vi "RETURN ITEM FRONT PANEL.vi"(9 "Main State":refnum<vi>, 10 "USER/ITEM DATA TRANSFER":refnum<vi>, 11 "RETURN ITEM":refnum<vi>) -> ()   [LabVIEW 2019]
uses:
  Controls/Table Data Types/Inventory Data Type.ctl
  <vilib>/addons/database/Auxilliary.llb/DB Tools Cursor Type.ctl
  Controls/Table Data Types/User Data Type.ctl
  Controls/State Variables/Main States.ctl
  Controls/Table Data Types/Checked In Archive Data Type.ctl
  Controls/Column Names/Inventory Column Names.ctl
  <vilib>/addons/database/Connection.llb/DB Tools Open Connec (String).vi
  <vilib>/addons/database/Connection.llb/Conn Execute.vi
  <vilib>/addons/database/Recordset.llb/Rec Fetch Recordset Data (R).vi
  <vilib>/addons/database/Recordset.llb/Rec Destroy - Connection.vi
  <vilib>/addons/database/_DB Variant To Data/Database Variant To Data.xnode
  <vilib>/addons/database/NI_Database_API.lvlib
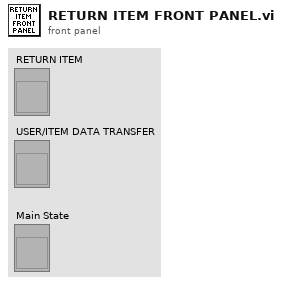
[diagram p1: front panel]
types:
  T1 = typedef "NI_Database_API.lvlib/DB Tools Cursor Type.ctl" = enum16{"forward-only", "keyset", "dynamic", "static"}
  T2 = typedef "Inventory Data Type.ctl" = cluster{"Identifier":string, "BYU ICN #":string, "Item Description":string, "Comments":string, "Checked Out Date":string, "Due Date":string, "Check Out Location":string, "Reminder Count":i32, "Most Recent Reminder Date":string, "BYU ID #":string, "Building/Room":string, "Location in Room":string, "Manual":string, "Manufacturer":string, "Model #":string, "Serial #":string, "Date Acquired":string}
  T3 = typedef "User Data Type.ctl" = cluster{"BYU ID #":string, "First Name":string, "Last Name":string, "Phone Number":string, "Email":string, "Department":string, "Graduation Status":string, "Anticipated Graduation Year":string, "Credit Score":dbl, "Date Added":string, "Graduation Clearance Date":string, "Picture File Name":string, "User Comments":string}
  T4 = typedef "Main States.ctl" = enum16{"INIT", "IDLE", "ADD USER", "EDIT USER", "ADD ITEM", "EDIT ITEM", "RETURN ITEMS", "SEARCH DATABASE", "USER ITEMS", "EDIT ITEMS", "CHECK OUT ITEMS", "TRANSFER ITEMS", "PSC SALES", "ATRIUM", "INVENTORY TRACKING", "SETTINGS", "REMINDER EMAILS", "END"}
  T5 = cluster{"DATA TYPE":enum16{"BYU ID", "ME#/IDENTIFIER", "BYU ICN"}, "DATA":string}
  T6 = typedef "Inventory Column Names.ctl" = string[]
  T7 = typedef "Checked In Archive Data Type.ctl" = cluster{"Identifier":string, "BYU ICN #":string, "Item Description":string, "Comments":string, "Checked Out Date":string, "Due Date":string, "Check Out Location":string, "Reminder Count":i32, "Most Recent Reminder Date":string, "BYU ID #":string, "Building/Room":string, "Location in Room":string, "Manual":string, "Manufacturer":string, "Model #":string, "Serial #":string, "Date Acquired":string, "Date Returned":string}
  T8 = typedef "NI_Database_API.lvlib/Conn ObjectReference.ctl" = refnum<k1>
  T9 = typedef "NI_Database_API.lvlib/Rec ObjectReference.ctl" = refnum<k1>
  T10 = cluster{"DATA TYPE":enum16{"BYU ID", "ME#/IDENTIFIER", "BYU ICN"}, "DATA":string}[]
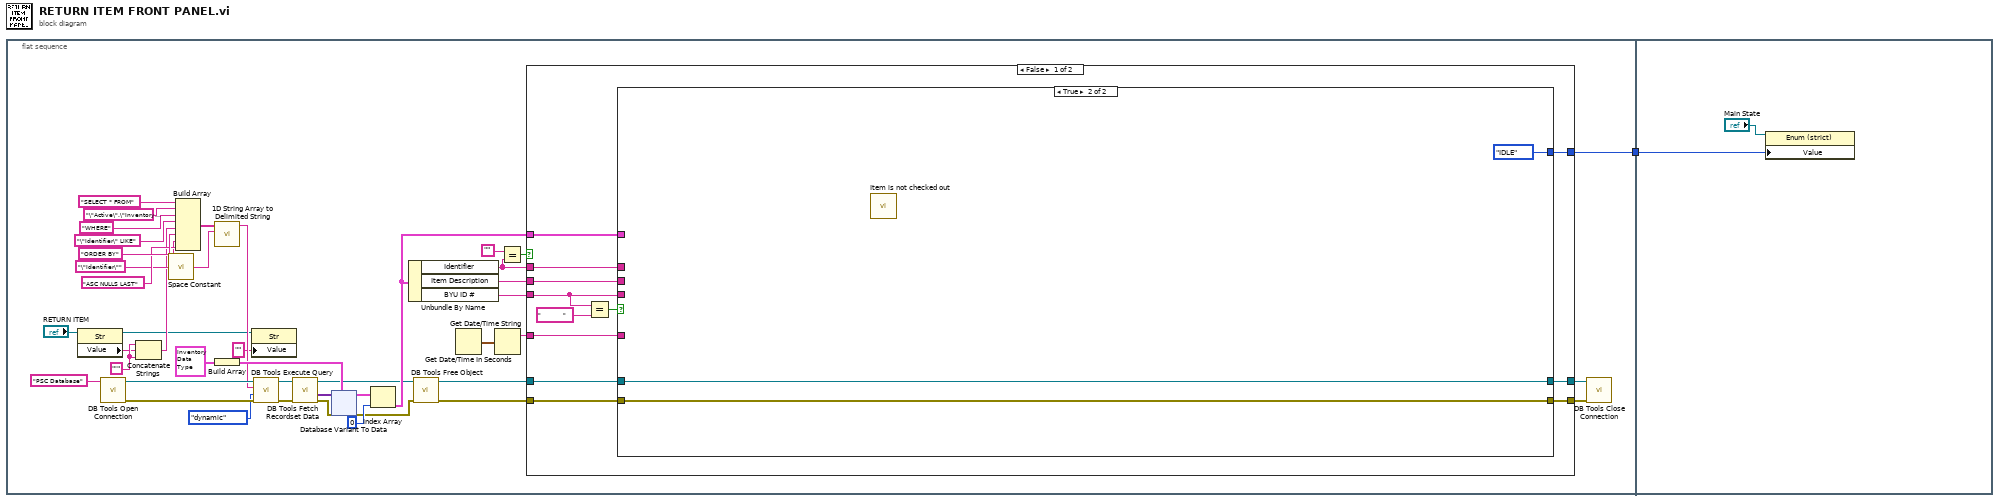
[diagram p0: block diagram]
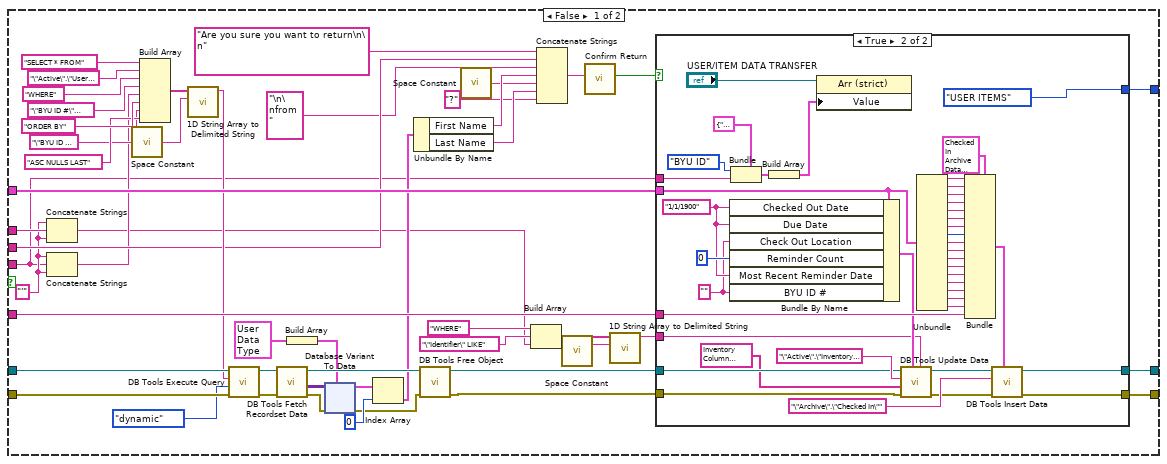
[diagram p2: hidden frame]
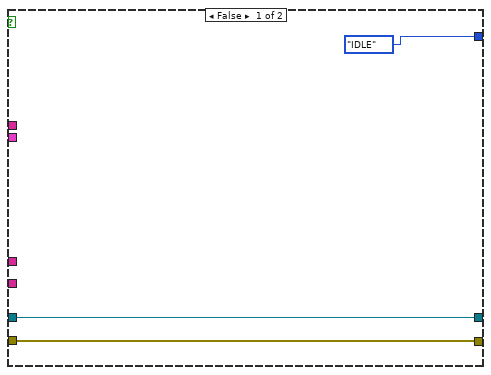
[diagram p3: hidden frame]
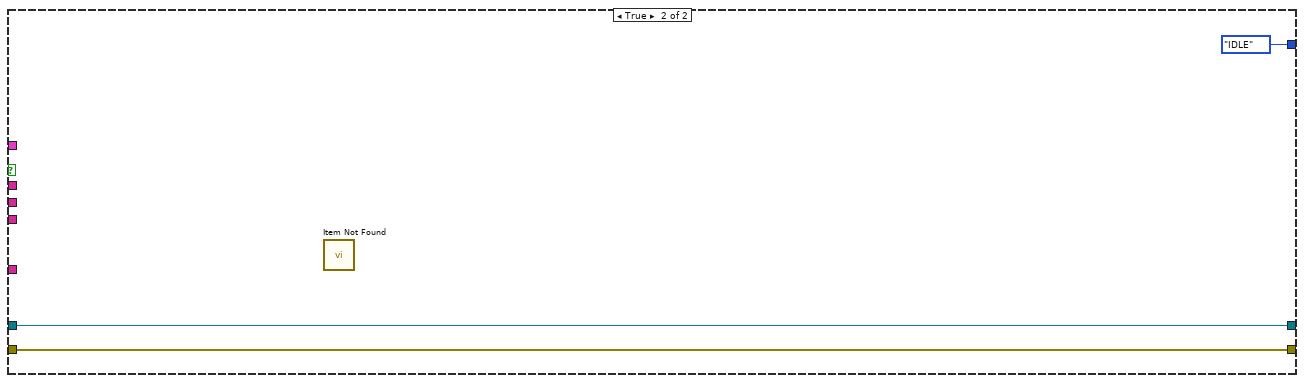
[diagram p4: hidden frame]
diagram:
  n1 = flat-sequence {
    tunnel: [w2] -> w1
    tunnel: w1 -> [w1108]
    frame #0 {
      w18 = "'" ("string")
      n2 = property class="Str"(reference="RETURN ITEM") -> (reference out=w4:refnum<vi>, "Value"=w16:string)  [unwired: 1 in, 1 out]
      n3 = call-poly <vilib>:"DB Tools Open Connection.vi"("connection information"="PSC Database") -> ("error out"=w42:errorcluster, "connection reference"=w43:T8)  [unwired: 7 in]
      n4 = Concatenate Strings(w18, w16, w18) -> (w17:string)
      n5 = call <vilib>:"Space Constant.vi"() -> ("String"=w32:string)
      n6 = Build Array("SELECT * FROM" ("SQL query"), "\"Active\".\"Inventory\"", "WHERE", "\"Identifier\" LIKE" ("string"), w17, "ORDER BY" ("string"), "\"Identifier\"" ("string"), "ASC NULLS LAST") -> (w31:string[])
      n7 = call <vilib>:"1D String Array to Delimited String.vi"("delimiter"=w32, "string array"=w31) -> ("delimited string"=w24:string)  [unwired: 9 in]
      n8 = Build Array(T2 {"Identifier"="", "BYU ICN #"="", "Item Description"="", "Comments"="", "Checked Out Date"="", "Due Date"="", "Check Out Location"="", "Reminder Count"=0, "Most Recent Reminder Date"="", "BYU ID #"="", "Building/Room"="", "Location in Room"="", "Manual"="", "Manufacturer"="", "Model #"="", "Serial #"="", "Date Acquired"=""} ("Array")) -> (w33:T2[])
      n9 = property class="Str"(reference=w4, "Value"="") -> ()  [unwired: 1 in, 2 out]
      n10 = call-poly <vilib>:"DB Tools Execute Query.vi"("error in (no error)"=w42, "cursor type"=DB_Tools_Cursor_Type."dynamic", "SQL query"=w24, "connection reference"=w43) -> ("error out"=w23:errorcluster, "recordset reference"=w22:T9)  [unwired: 4 in]
      n11 = call-poly <vilib>:"DB Tools Fetch Recordset Data.vi"("error in (no error)"=w23, "recordset reference"=w22) -> ("error out"=w20:errorcluster, "recordset data"=w21:variant[][], "recordset reference out"=w10:T9)  [unwired: 3 in]
      n12 = xnode "Database Variant To Data"("database variant"=w21, "error in (no error)"=w20, "type"=w33) -> ("data"=w36:T2[], "error out"=w9:errorcluster)
      n13 = Index Array(array=w36, index=0) -> (element=w15:T2)
      n14 = Unbundle By Name(w15) -> ("Identifier"=w5:string, "Item Description"=w12:string, "BYU ID #"=w11:string)
      n15 = call-poly <vilib>:"DB Tools Free Object.vi"("error in (no error)"=w9, "recordset reference"=w10) -> ("error out"=w7:errorcluster, "connection reference"=w8:T8)  [unwired: 8 in]
      n16 = Get Date/Time In Seconds() -> (seconds since 1Jan1904=w40:timestamp)
      n17 = Get Date/Time String(seconds (now)=w40) -> (date string=w37:string)  [unwired: 2 in, 1 out]
      n18 = Equal?(x="", y=w5) -> (x = y?=w13:bool)
      n19 = case shown="False" w13 {
        tunnel: [w56 w570] -> w39
        tunnel: [w55 w569] -> w38
        tunnel: w37 -> [w54 _]
        tunnel: w15 -> [w53 _]
        tunnel: w12 -> [w50 _]
        tunnel: w11 -> [w48 _]
        tunnel: w8 -> [w52 w570]
        tunnel: w7 -> [w51 w569]
        tunnel: w5 -> [w49 _]
        tunnel: [w46 Main_States."IDLE" ("Value")] -> w2
        frame False {
          n20 = Equal?(x=w48, y="           ") -> (x = y?=w47:bool)
          n21 = case shown="True" w47 {
            tunnel: [w106 w567] -> w56
            tunnel: [w105 w566] -> w55
            tunnel: w54 -> [w104 _]
            tunnel: w53 -> [w103 _]
            tunnel: w52 -> [w85 w567]
            tunnel: w51 -> [w84 w566]
            tunnel: w50 -> [w77 _]
            tunnel: w49 -> [w64 _]
            tunnel: w48 -> [w58 _]
            tunnel: [w57 Main_States."IDLE" ("Value")] -> w46
            frame False {
              w63 = "'" ("string")
              n22 = Concatenate Strings(w63, w64, w63) -> (w61:string)
              n23 = Concatenate Strings(w63, w58, w63) -> (w62:string)
              n24 = call <vilib>:"Space Constant.vi"() -> ("String"=w102:string)
              n25 = Build Array("SELECT * FROM" ("SQL query"), "\"Active\".\"Users\"", "WHERE", "\"BYU ID #\" LIKE" ("string"), w62, "ORDER BY" ("string"), "\"BYU ID #\"" ("string"), "ASC NULLS LAST") -> (w101:string[])
              n26 = call <vilib>:"1D String Array to Delimited String.vi"("delimiter"=w102, "string array"=w101) -> ("delimited string"=w83:string)  [unwired: 9 in]
              n27 = call-poly <vilib>:"DB Tools Execute Query.vi"("error in (no error)"=w84, "cursor type"=DB_Tools_Cursor_Type."dynamic", "SQL query"=w83, "connection reference"=w85) -> ("error out"=w91:errorcluster, "recordset reference"=w90:T9)  [unwired: 4 in]
              n28 = call-poly <vilib>:"DB Tools Fetch Recordset Data.vi"("error in (no error)"=w91, "recordset reference"=w90) -> ("error out"=w88:errorcluster, "recordset data"=w89:variant[][], "recordset reference out"=w87:T9)  [unwired: 3 in]
              n29 = Build Array(T3 {"BYU ID #"="", "First Name"="", "Last Name"="", "Phone Number"="", "Email"="", "Department"="", "Graduation Status"="", "Anticipated Graduation Year"="", "Credit Score"=0.0, "Date Added"="", "Graduation Clearance Date"="", "Picture File Name"="", "User Comments"=""} ("USER DATA TYPE")) -> (w80:T3[])
              n30 = xnode "Database Variant To Data"("database variant"=w89, "error in (no error)"=w88, "type"=w80) -> ("data"=w93:T3[], "error out"=w86:errorcluster)
              n31 = Index Array(array=w93, index=0) -> (element=w79:T3)
              n32 = Unbundle By Name(w79) -> ("First Name"=w75:string, "Last Name"=w73:string)
              n33 = call-poly <vilib>:"DB Tools Free Object.vi"("error in (no error)"=w86, "recordset reference"=w87) -> ("error out"=w59:errorcluster, "connection reference"=w60:T8)  [unwired: 8 in]
              n34 = call <vilib>:"Space Constant.vi"() -> ("String"=w74:string)
              n35 = Build Array("WHERE", "\"Identifier\" LIKE" ("string"), w61) -> (w67:string[])
              n36 = Concatenate Strings("Are you sure you want to return\n\n" ("string"), w77, "\n\nfrom " ("string"), w75, w74, w73, "?" ("string")) -> (w71:string)
              n37 = call <vilib>:"Space Constant.vi"() -> ("String"=w66:string)
              n38 = call "Confirm Return"("Message"=w71) -> ("Yes, Return it"=w70:bool)  [unwired: 9 in, 1 out]
              n39 = call <vilib>:"1D String Array to Delimited String.vi"("delimiter"=w66, "string array"=w67) -> ("delimited string"=w65:string)  [unwired: 9 in]
              n40 = case shown="True" w70 {
                tunnel: [w109 w151] -> w106
                tunnel: [w108 w150] -> w105
                tunnel: w104 -> [_ w149]
                tunnel: w103 -> [_ w123]
                tunnel: w65 -> [_ w122]
                tunnel: w60 -> [w109 w121]
                tunnel: w59 -> [w108 w120]
                tunnel: w58 -> [_ w114]
                tunnel: [Main_States."IDLE" ("Value") Main_States."USER ITEMS" ("Value")] -> w57
                frame False {
                }
                frame True {
                  w117 = "" ("Checked Out Date")
                  w118 = "1/1/1900" ("Checked Out Date")
                  n41 = Bundle By Name(cluster=w123, "Checked Out Date"=w118, "Due Date"=w118, "Check Out Location"=w117, "Reminder Count"=0, "Most Recent Reminder Date"=w118, "BYU ID #"=w117) -> (w132:T2)
                  n42 = Bundle(cluster=T5 {"DATA TYPE"=enum."BYU ID", "DATA"=""} ("USER/ITEM DATA TRANSFER"), "DATA TYPE"=enum16{"BYU ID", "ME#/IDENTIFIER", "BYU ICN"}."BYU ID", "DATA"=w114) -> (w112:T5)
                  n43 = Build Array(w112) -> (w111:T10)
                  n44 = property class="Arr (strict)"(reference="USER/ITEM DATA TRANSFER", "Value"=w111) -> ()  [unwired: 1 in, 2 out]
                  n45 = call <vilib>:"DB Tools Update Data.vi"("condition"=w122, "data"=w132, "error in (no error)"=w120, "columns"=T6 ["\"Identifier\"", "\"BYU ICN #\"", "\"Item Description\"", "\"Comments\"", "\"Checked Out Date\"", "\"Due Date\"", "\"Check Out Location\"", "\"Reminder Count\"", "\"Most Recent Reminder Date\"", "\"BYU ID #\"", "\"Building/Room\"", "\"Location in Room\"", "\"Manual\"", "\"Manufacturer\"", "\"Model #\"", "\"Serial #\"", "\"Date Acquired\""] ("INVENTORY COLUMN NAMES"), "table"="\"Active\".\"Inventory\"", "connection reference"=w121) -> ("error out"=w144:errorcluster, "connection reference out"=w145:T8)  [unwired: 4 in]
                  n46 = Unbundle(w123) -> ("Identifier"=w142:string, "BYU ICN #"=w141:string, "Item Description"=w140:string, "Comments"=w139:string, "Checked Out Date"=w138:string, "Due Date"=w137:string, "Check Out Location"=w136:string, "Reminder Count"=w135:i32, "Most Recent Reminder Date"=w134:string, "BYU ID #"=w133:string, "Building/Room"=w125:string, "Location in Room"=w126:string, "Manual"=w127:string, "Manufacturer"=w128:string, "Model #"=w129:string, "Serial #"=w130:string, "Date Acquired"=w131:string)
                  n47 = Bundle(cluster=T7 {"Identifier"="", "BYU ICN #"="", "Item Description"="", "Comments"="", "Checked Out Date"="", "Due Date"="", "Check Out Location"="", "Reminder Count"=0, "Most Recent Reminder Date"="", "BYU ID #"="", "Building/Room"="", "Location in Room"="", "Manual"="", "Manufacturer"="", "Model #"="", "Serial #"="", "Date Acquired"="", "Date Returned"=""} ("CHECKED IN ARCHIVE DATA TYPE"), "Identifier"=w142, "BYU ICN #"=w141, "Item Description"=w140, "Comments"=w139, "Checked Out Date"=w138, "Due Date"=w137, "Check Out Location"=w136, "Reminder Count"=w135, "Most Recent Reminder Date"=w134, "BYU ID #"=w133, "Building/Room"=w125, "Location in Room"=w126, "Manual"=w127, "Manufacturer"=w128, "Model #"=w129, "Serial #"=w130, "Date Acquired"=w131, "Date Returned"=w149) -> (w147:T7)
                  n48 = call <vilib>:"DB Tools Insert Data.vi"("data"=w147, "error in (no error)"=w144, "table"="\"Archive\".\"Checked In\"", "connection reference"=w145) -> ("error out"=w150:errorcluster, "connection reference out"=w151:T8)  [unwired: 6 in]
                }
              }
            }
            frame True {
              n49 = call "Item is not checked out"() -> ()  [unwired: 10 in, 2 out]
            }
          }
        }
        frame True {
          n50 = call "Item Not Found"() -> ()  [unwired: 10 in, 2 out]
        }
      }
      n51 = call <vilib>:"DB Tools Close Connection.vi"("error in (no error)"=w38, "connection reference"=w39) -> ()  [unwired: 5 in, 1 out]
    }
    frame #1 {
      n52 = property class="Enum (strict)"(reference="Main State", "Value"=w1108) -> ()  [unwired: 1 in, 2 out]
    }
  }
